vi "ObtainQueueMainController.vi"(8 "error in (no error)":errorcluster) -> (0 "error out":errorcluster, 3 "MainQueue":refnum<queue>)   [LabVIEW 2019, in "MainController.lvlib"]
uses:
  MainController.lvlib
  Cluster - MainControllerMessage.ctl
  Enum - MainState.ctl
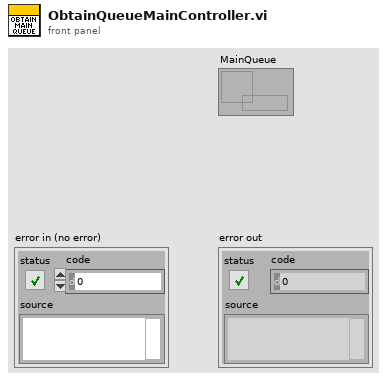
[diagram p1: front panel]
types:
  T1 = typedef "MainController.lvlib/Cluster - MainControllerMessage.ctl" = cluster{"Message":T2, "Data":variant}
  T2 = typedef "MainController.lvlib/Enum - MainState.ctl" = enum16{"Initialize", "InitUIRefs", "LaunchSettings", "LaunchAutoMode", "LaunchManualMode", "LaunchTestReport", "ConnectHardware", "DisconnectHardware", "HiliteNavItems", "StartAutoMode", "PauseAutoMode", "StopAutoMode", "ShowFlyout", "HideFlyout", "BroadcastSettings", "PickupTestSettings", "BroadcastHW", "AutoTestDone", "DAQStatus", "UpdateCommandBar", "Error", "RecieveError", "Exit"}
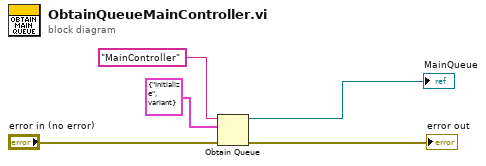
[diagram p0: block diagram]
diagram:
  n1 = Obtain Queue(name (unnamed)="MainController", element data type=T1 {"Message"=enum."Initialize", "Data"=variant}, error in (no error)="error in (no error)") -> (queue out=→"MainQueue":refnum<queue>, error out=→"error out":errorcluster)  [unwired: 2 in, 1 out]
